vi "LABVEIW_project_Tramitter.vi"() -> ()   [LabVIEW 2020]
uses:
  <vilib>/measure/maspectr.llb/FFT Power Spectrum and PSD for 1 Chan.vi
  <instrlib>/niUSRP/niUSRP Write Tx Data (CDB WDT).vi
  <vilib>/measure/NI_MABase.lvlib
  <vilib>/measure/NI_MAPro.lvlib
panel:
  out "Transmiting Signal":dbl[](graph)
  in  "stop":bool
  in  "frequency":dbl=10.0 format="%0.2p"
  in  "signal type":T1(ring)
  in  "amplitude":dbl=1.0 format="%0.2p"
  out "Original Signal":waveform(dbl)(graph)
  in  "standard deviation":dbl=1.0 format="%.2p"
  out "Signal with noise":waveform(dbl)(graph)
  out "psd of signal with noise":cluster{"f0":dbl, "df":dbl, "magnitude":dbl[]}(graph)
  out "Filtered signal":dynamicdata(graph)
  in  "gain":dbl format="%#_6f"
  in  "carrier frequency":dbl=100000.0 format="%#_6p"
  in  "IQ rate":dbl=100000.0 format="%#_6p"
  in  "active antenna":string
  in  "device names":refnum<k15>
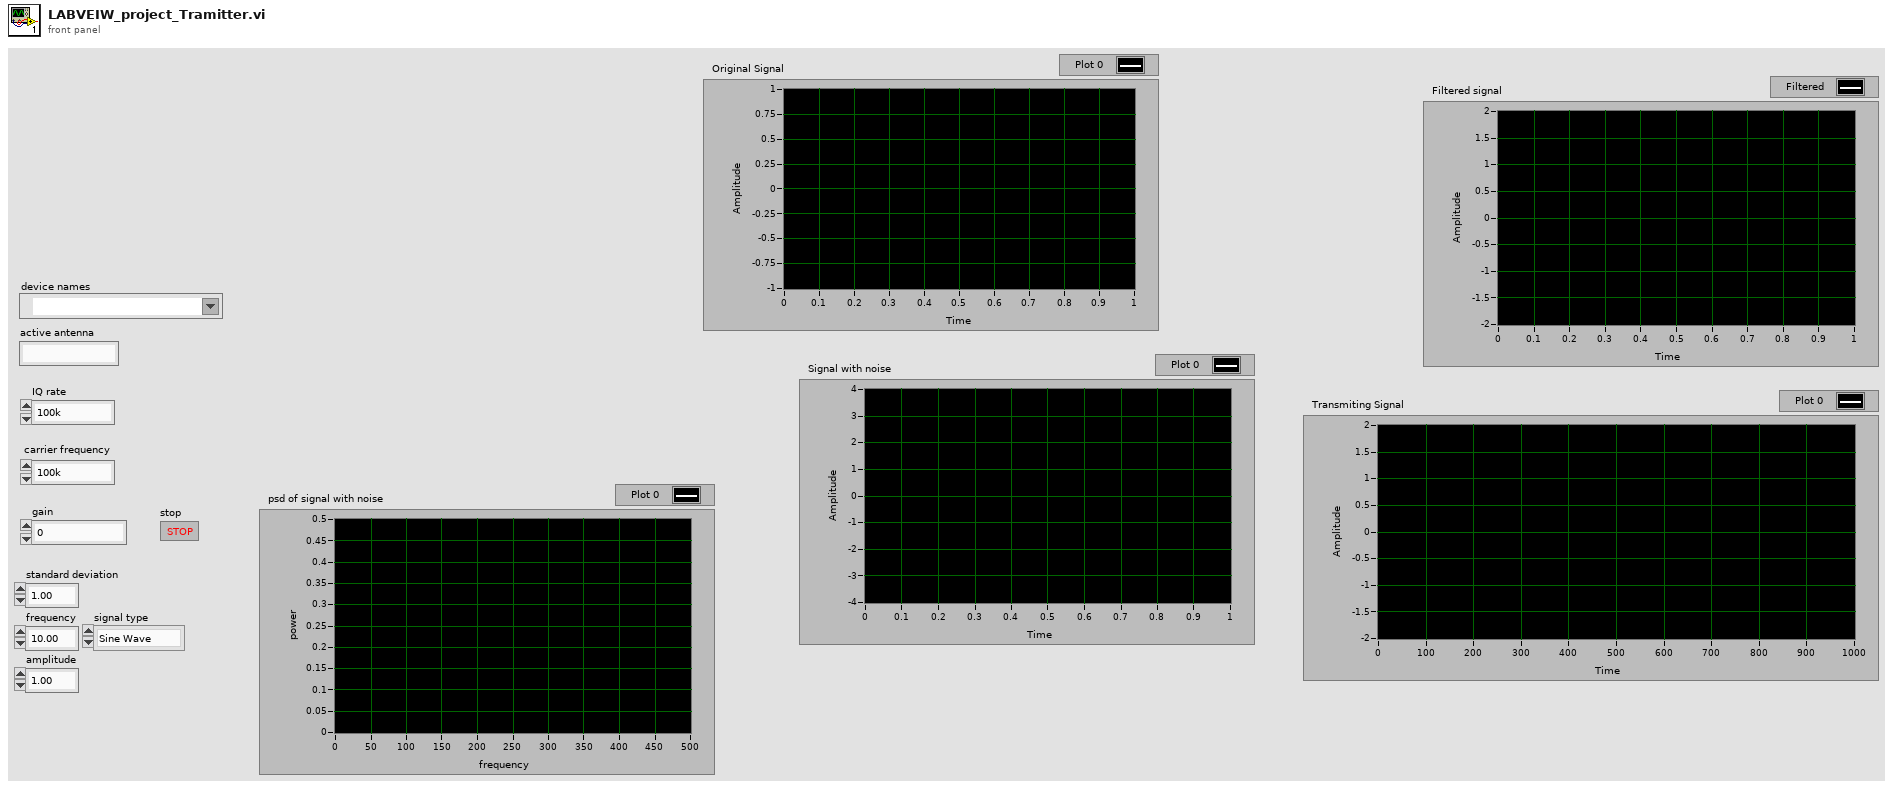
[diagram p1: front panel]
types:
  T1 = enum16{"Sine Wave", "Triangle Wave", "Square Wave", "Sawtooth Wave"}
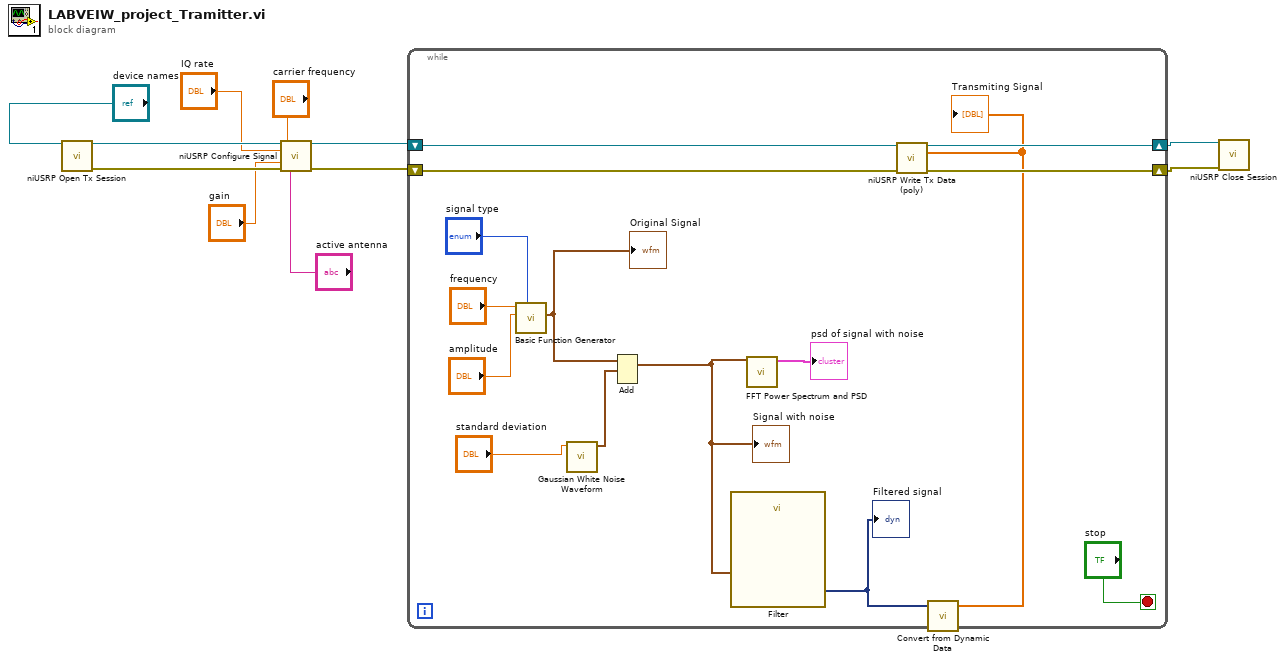
[diagram p0: block diagram]
diagram:
  n1 = call <instrlib>:"niUSRP Open Tx Session.vi"("device names"="device names") -> ("session handle out"=w11:refnum<k15>, "error out"=w8:errorcluster)  [unwired: 13 in]
  n2 = call <instrlib>:"niUSRP Configure Signal.vi"("session handle"=w11, "IQ rate"="IQ rate", "carrier frequency"="carrier frequency", "gain"="gain", "error in (no error)"=w8, "active antenna"="active antenna") -> ("session handle out"=w10:refnum<k15>, "error out"=w7:errorcluster)  [unwired: 5 in, 3 out]
  n3 = while {
    shift-right: [w25] -> w9
    shift-left: w10 -> [w26]
    shift-right: [w23] -> w6
    shift-left: w7 -> [w24]
    stop <- "stop" stop-if-true
    n4 = call <vilib>:"Basic Function Generator.vi"("signal type"="signal type", "amplitude"="amplitude", "frequency"="frequency") -> ("signal out"=w17:waveform(dbl))  [unwired: 6 in, 2 out]
    "Original Signal" <- w17
    n5 = call <vilib>:"Gaussian White Noise Waveform.vi"("standard deviation"="standard deviation") -> ("signal out"=w16:waveform(dbl))  [unwired: 9 in, 1 out]
    n6 = Add(1:w16, 2:w17) -> (0:w14:waveform(dbl))  [unwired: 1 in, 1 out]
    "Signal with noise" <- w14
    n7 = call "Filter"("Signal"=w14) -> ("Filtered Signal"=w13:dynamicdata)  [unwired: 9 in, 1 out]
    "Filtered signal" <- w13
    n8 = call-poly <vilib>:"FFT Power Spectrum and PSD.vi"("time signal"=w14) -> ("Power Spectrum / PSD"=→"psd of signal with noise":cluster{"f0":dbl, "df":dbl, "magnitude":dbl[]})  [unwired: 7 in, 3 out]
    n9 = call "Convert from Dynamic Data"("Dynamic Data Type"=w13) -> ("Array"=w12:dbl[])  [unwired: 3 in]
    "Transmiting Signal" <- w12
    n10 = call-poly <instrlib>:"niUSRP Write Tx Data (poly).vi"("session handle"=w26, "data"=w12, "error in (no error)"=w24) -> ("session handle out"=w25:refnum<k15>, "error out"=w23:errorcluster)  [unwired: 11 in]
  }
  n11 = call <instrlib>:"niUSRP Close Session.vi"("session handle"=w9, "error in (no error)"=w6) -> ()  [unwired: 13 in, 1 out]
